vi "Pre Launch Init.vi"(11 "ConnectionFactoryHandler in":refnum<class "ConnectionFactoryHandler.lvclass">) -> (0 "error out":errorcluster, 3 "ConnectionFactoryHandler out":refnum<class "ConnectionFactoryHandler.lvclass">)   [LabVIEW 2020, in "ConnectionFactorySession.lvlib" / "ConnectionFactoryHandler.lvclass"]
doc: "(<B>Filename</B>: Actor Framework.lvlib:Actor.lvclass:Pre Launch Init.vi)\n\nDefines behavior that occurs after the Launch Nested Actor method is invoked but before the actor's Actor Core method begins running.\n\nBy default, this method does nothing. A descendant class may override it to define behavior."
uses:
  <vilib>/gpm_packages/@cs/Network-interface/Source/Connection Factory Session/ConnectionFactoryHandler/ConnectionFactoryHandler.lvclass
  <vilib>/gpm_packages/@cs/Network-interface/Source/Connection Factory Session/INewConnectionCallback/INewConnectionCallback.lvclass
  <vilib>/gpm_packages/@cs/Network-interface/Source/Connection Factory Session/ConnectionFactoryHandler/ConnectionFactoryHandler.lvclass/ConnectionFactoryHandler.ctl
  <vilib>/gpm_packages/@cs/Network-interface/Source/Logged Actor/LoggedActor.lvclass
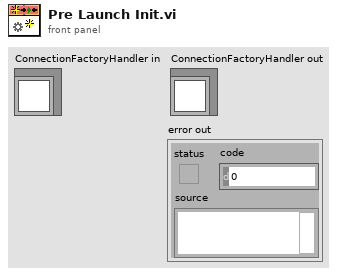
[diagram p1: front panel]
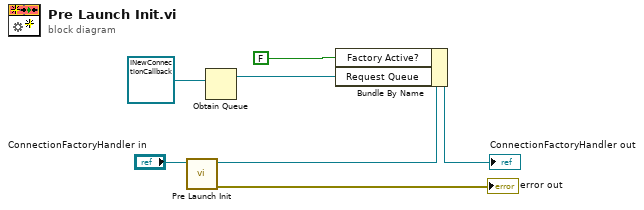
[diagram p0: block diagram]
diagram:
  n1 = call-parent "Pre Launch Init.vi"("Logged Actor in"="ConnectionFactoryHandler in") -> ("error out"=→"error out":errorcluster, "Logged Actor out"=w6:refnum<class "ConnectionFactoryHandler.lvclass">)  [unwired: 9 in]
  n2 = Obtain Queue(element data type=refnum<class "INewConnectionCallback.lvclass"> refnum ("Active Connection Request")) -> (queue out=w1:refnum<queue>)  [unwired: 4 in, 2 out]
  n3 = Bundle By Name(cluster=w6, "Factory Active?"=FALSE, "Request Queue"=w1) -> (→"ConnectionFactoryHandler out":refnum<class "ConnectionFactoryHandler.lvclass">)
